vi "ThermalVideoStream.vi"() -> ()   [LabVIEW 2022 SP3]
panel:
  in  "base path":path
  out "Image":T1(plugin-control)
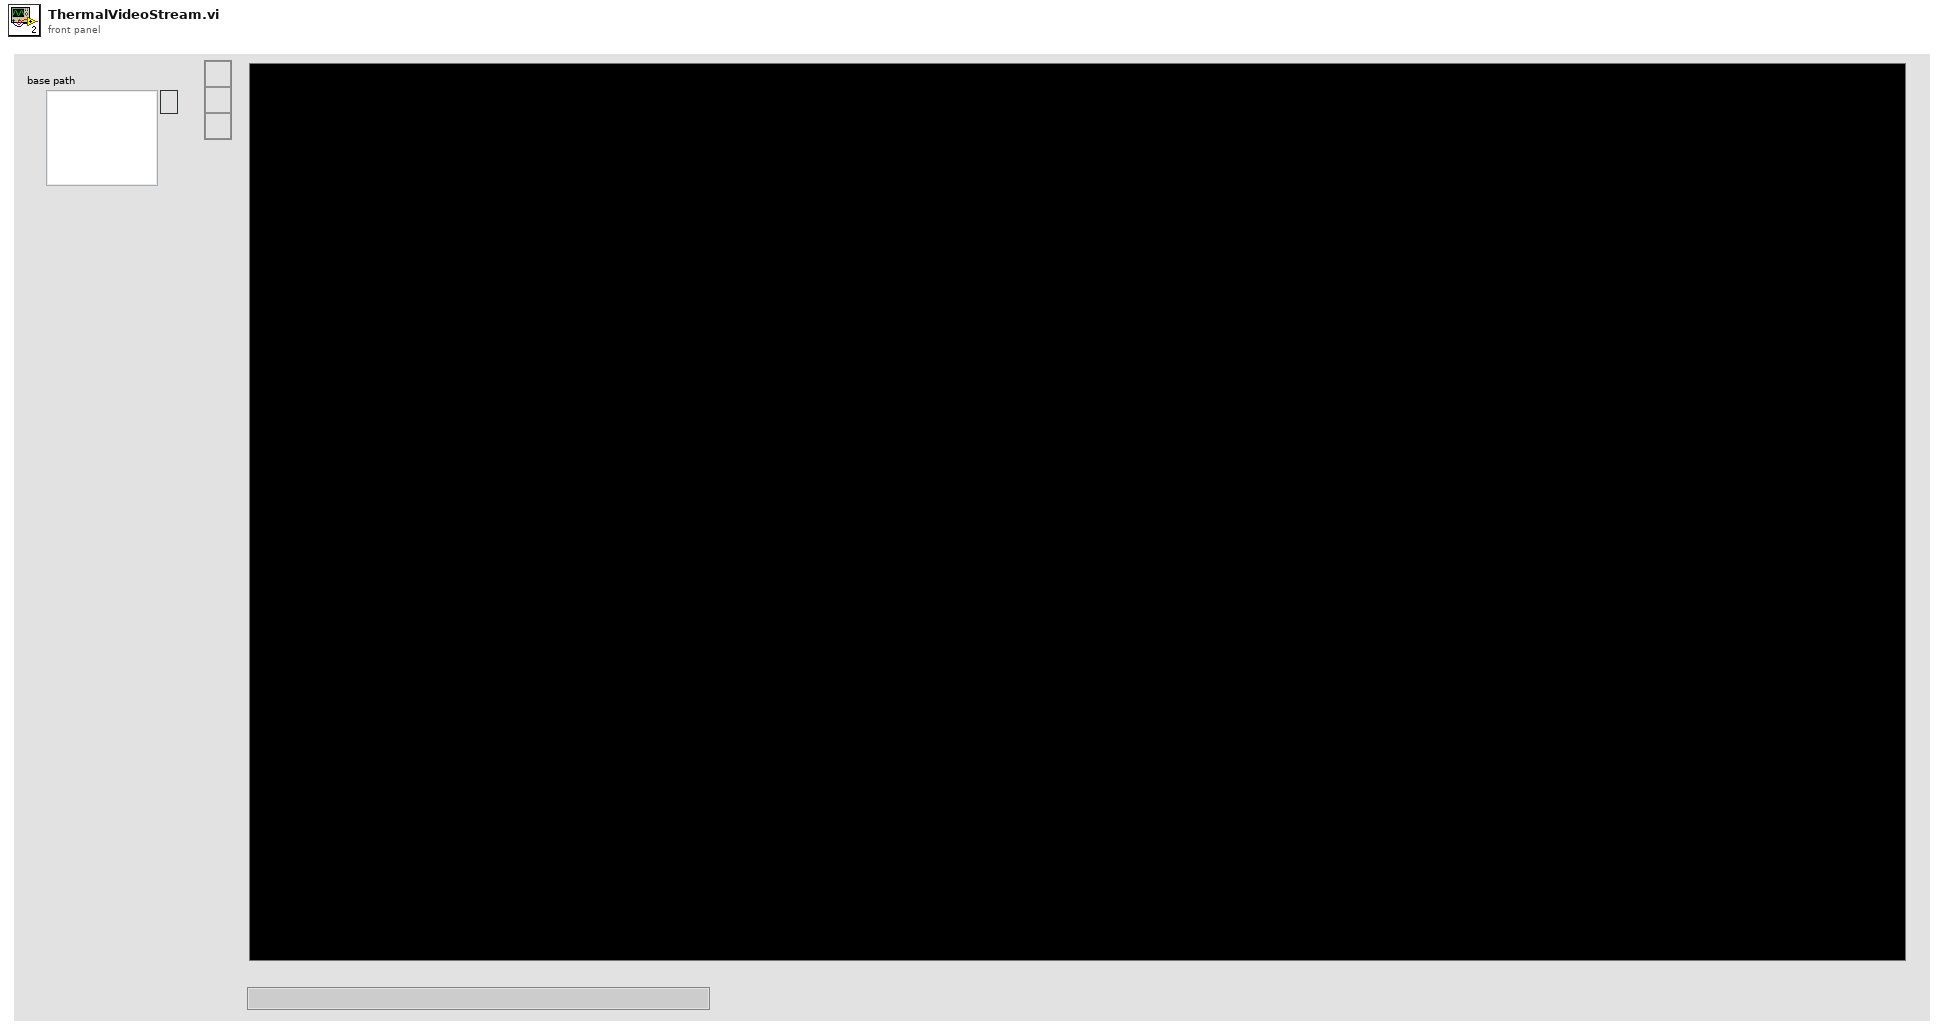
[diagram p1: front panel]
types:
  T1 = typedef "IMAQ Image.ctl" = refnum<image>
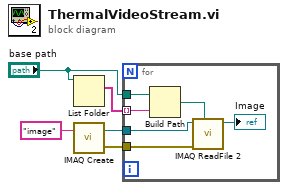
[diagram p0: block diagram]
diagram:
  n1 = List Folder(path="base path") -> (filenames=w3:string[])  [unwired: 3 in, 3 out]
  n2 = call "IMAQ Create"("Image Name"="image") -> ("New Image"=w4:T1, "error out"=w5:errorcluster)  [unwired: 4 in]
  n3 = for {
    tunnel: w5 -> [w10]
    tunnel: w4 -> [w9]
    tunnel: w3 -> [w8] mode=indexing
    tunnel: "base path" -> [w7]
    n4 = Build Path(base path=w7, name or relative path=w8) -> (appended path=w11:path)
    n5 = call "IMAQ ReadFile 2"("File Path"=w11, "error in (no error)"=w10, "Image"=w9) -> ("Image Out"=→"Image":T1)  [unwired: 4 in, 4 out]
  }
